vi "EvaluationWaypoint.vi"(8 "error in (no error)":errorcluster, 10 "Parents G":dbl, 11 "Waypoint in":refnum<class "Waypoint.lvclass">) -> (0 "error out":errorcluster, 1 "H":dbl, 2 "G":dbl, 3 "Waypoint out":refnum<class "Waypoint.lvclass">)   [LabVIEW 2010, in "Waypoint.lvclass"]
uses:
  Waypoint.lvclass
  Waypoint.lvclass/Waypoint.ctl
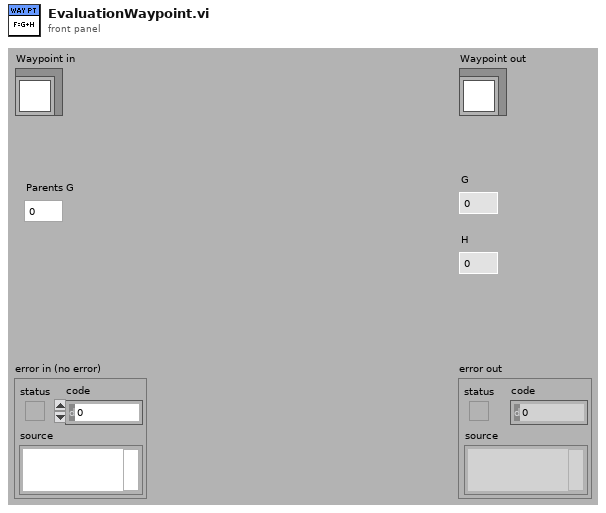
[diagram p1: front panel]
types:
  T1 = typedef "Waypoint.lvclass/point.ctl" = cluster{"X":dbl, "Y":dbl}
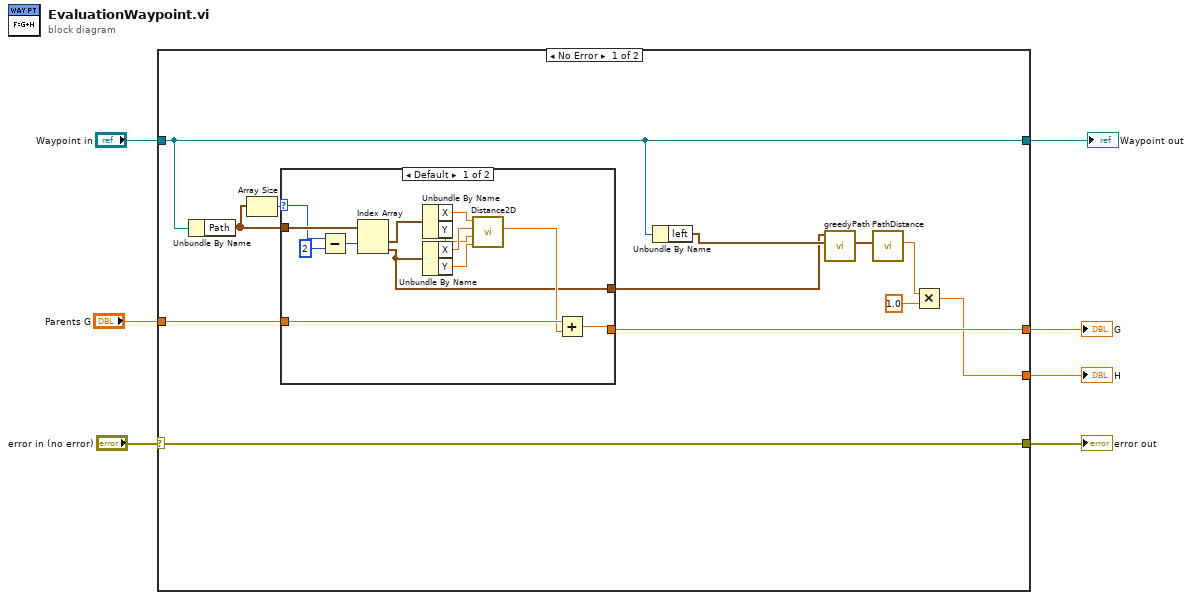
[diagram p0: block diagram]
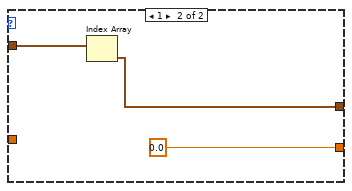
[diagram p2: hidden frame]
diagram:
  n1 = case shown="No Error" "error in (no error)" {
    selector: "error in (no error)" -> [w19 w37]
    tunnel: "Waypoint in" -> [w14 w36]
    tunnel: "Parents G" -> [w17 _]
    tunnel: [w16 _] -> w4
    tunnel: [w8 _] -> w3
    tunnel: [w19 w37] -> w2
    tunnel: [w14 w36] -> w1
    frame No Error {
      n2 = Unbundle By Name(w14) -> ("Path"=w15:T1[])
      n3 = Array Size(array=w15) -> (size(s)=w18:i32)
      n4 = case shown="Default" w18 {
        selector: w18 -> [w31 _]
        tunnel: w17 -> [w23 _]
        tunnel: [w21 0.0] -> w16
        tunnel: w15 -> [w32 w34]
        tunnel: [w20 w33] -> w12
        frame Default {
          n5 = Subtract(x=w31, y=2) -> (x-y=w29:i32)
          n6 = Index Array(array=w32, index #1=w29) -> (element #1=w28:T1, element #2=w20:T1)  [unwired: 1 in]
          n7 = Unbundle By Name(w28) -> ("X"=w27:dbl, "Y"=w25:dbl)
          n8 = Unbundle By Name(w20) -> ("X"=w26:dbl, "Y"=w24:dbl)
          n9 = call "Distance2D.vi"("y2"=w24, "y1"=w25, "x2"=w26, "x1"=w27) -> ("distance"=w22:dbl)  [unwired: 7 in]
          n10 = Add(x=w23, y=w22) -> (x+y=w21:dbl)
        }
        frame 1 {
          n11 = Index Array(array=w34) -> (element=w33:T1)  [unwired: 1 in]
        }
      }
      n12 = Unbundle By Name(w14) -> ("left"=w13:T1[])
      n13 = call "greedyPath.vi"("ToVisit"=w13, "start"=w12) -> ("greedy Path"=w11:T1[])  [unwired: 8 in, 1 out]
      n14 = call "PathDistance.vi"("path"=w11) -> ("distance"=w10:dbl)  [unwired: 10 in]
      n15 = Multiply(x=w10, y=1.0) -> (x*y=w8:dbl)
    }
    frame Error {
    }
  }
  "error out" <- w2
  "Waypoint out" <- w1
  "G" <- w4
  "H" <- w3
